vi "Read Grating ID.vi"(8 "error in (no error)":errorcluster, 11 "VISA resource name":refnum<visa-resource-name>) -> (0 "error out":errorcluster, 2 "Grating ID":i32, 3 "VISA resource name out":refnum<visa-resource-name>, 4 "read buffer":string)   [LabVIEW 2019, in "SpectraPro.lvlib"]
uses:
  SpectraPro.lvlib
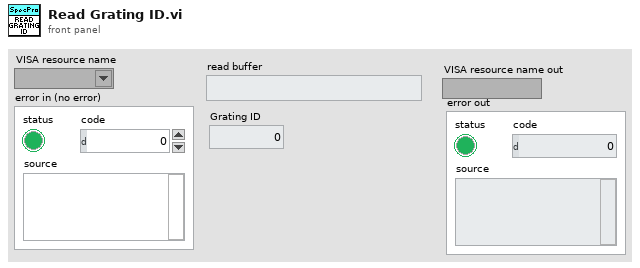
[diagram p1: front panel]
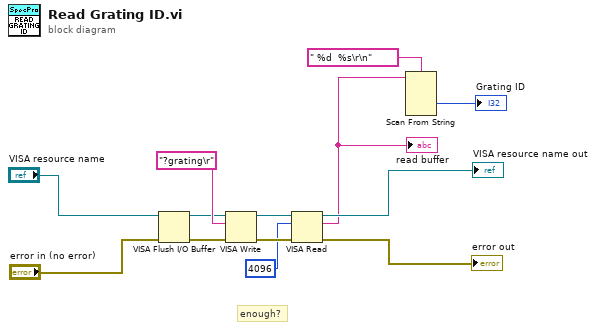
[diagram p0: block diagram]
diagram:
  # "enough?"
  n1 = VISA Flush I/O Buffer(VISA resource name="VISA resource name", error in (no error)="error in (no error)") -> (VISA resource name out=w6:refnum<visa-resource-name>, error out=w7:errorcluster)  [unwired: 1 in]
  n2 = VISA Write(VISA resource name=w6, write buffer="?grating\r", error in (no error)=w7) -> (VISA resource name out=w10:refnum<visa-resource-name>, error out=w11:errorcluster)  [unwired: 1 out]
  n3 = VISA Read(VISA resource name=w10, byte count=u32 4096, error in (no error)=w11) -> (VISA resource name out=→"VISA resource name out":refnum<visa-resource-name>, read buffer=w3:string, error out=→"error out":errorcluster)  [unwired: 1 out]
  "read buffer" <- w3
  n4 = Scan From String(format string=" %d  %s\r\n", input string=w3) -> (output 1=→"Grating ID":i32)  [unwired: 5 in, 3 out]
